vi "XIPIN_DMA_Subsystem_for_PCI_Express_(PCIe)_1_0.vi"   [LabVIEW 2017]
doc: "The Xilinx PCI Express DMA\n------------------------------------\n<b>Need License</b> : Yes\n<b>Interface</b> : AXI4 AXI4-Stream"
uses:
  <vilib>/rvi/XilinxIP/XIPIN_XNode/niFpgaXIPIN.xnode
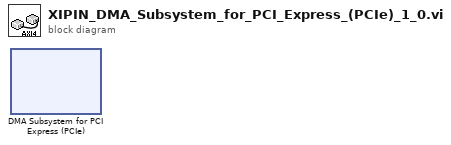
[diagram p0: block diagram]
diagram:
  n1 = xnode ("DMA Subsystem for PCI Express (PCIe)")() -> ()
